vi "Autonomous Independent.vi"() -> ()   [LabVIEW 2013]
doc: "This VI is called when autonomous begins, and will automatically be terminated when autonomous ends. You can carry out timed or sensor driven robot movement independently without needing to return to the caller."
uses:
  <vilib>/Rock Robotics/WPI/Joystick/WPI_JoystickAxis.ctl
  Robot Global Data.vi
  <vilib>/Rock Robotics/WPI/Joystick/WPI_JoystickGetSetRefNum.vi
  <vilib>/Rock Robotics/WPI/RobotDrive/WPI_RobotDriveArcadeDrive_Standard(NoSaturation).vi
panel:
  out "Current Movement, for debugging":T1 {"Y Joystick Value" scale=1.0..-1.0; "X Joystick Value" scale=-1.0..1.0}
  in  "Array of robot movements":T2(array[cluster]) {"Y Joystick Value" scale=1.0..-1.0; "X Joystick Value" scale=-1.0..1.0}
  # "Be sure to right-click and choose Data Operations>>Make Current Value default if you want to save the array values with the VI"
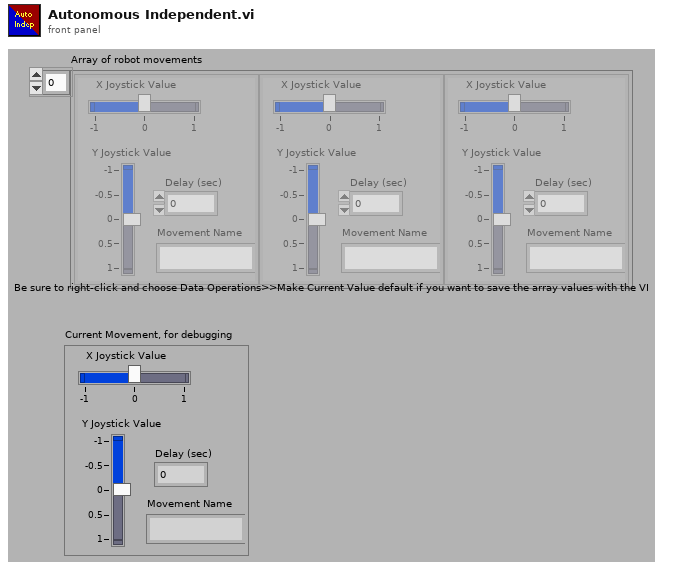
[diagram p1: front panel]
types:
  T1 = cluster{"X Joystick Value":dbl, "Y Joystick Value":dbl, "Delay (sec)":dbl, "Movement Name":string}
  T2 = cluster{"X Joystick Value":dbl, "Y Joystick Value":dbl, "Delay (sec)":dbl, "Movement Name":string}[]
  T3 = typedef "WPI_JoystickAxis.ctl" = enum16{"Axis 1", "Axis 2", "Axis 3", "Axis 4", "Axis 5", "Axis 6"}
  T4 = typedef "WPI_JoystickDevRef.ctl" = cluster{"Device":T5}
  T5 = typedef "WPI_JoystickDeviceEnum.ctl" = enum16{"USB 1", "USB 2", "USB 3", "USB 4", "Kinect 1", "Kinect 2"}
  T6 = typedef "WPI_ServoDeviceRef.ctl" = cluster{"DeviceStatus":errorcluster, "Digital Module":T7, "PWM Channel":T8, "DeadBand":T9}
  T7 = typedef "FPGA_TypedefDigitalModule.ctl" = enum16{"Digital Module 1", "Digital Module 2"}
  T8 = typedef "FPGA_DIOPWMChannel.ctl" = enum8{"PWM 1", "PWM 2", "PWM 3", "PWM 4", "PWM 5", "PWM 6", "PWM 7", "PWM 8", "PWM 9", "PWM 10", "Invalid"}
  T9 = typedef "WPI_PWMDeadband.ctl" = cluster{"Name":string, "maxPositivePwm":i32, "minPositivePwm":i32, "centerPwm":i32, "maxNegativePwm":i32, "minNegativePwm":i32, "angularRange":u16}
  T10 = typedef "WPI_MotorControlDeviceRef.ctl" = cluster{"DeviceStatus":errorcluster, "Type":enum16{"PWM", "CAN"}, "PWM":cluster{"Digital Module":T7, "PWM Channel":T8, "DeadBand":T9}, "CAN":cluster{"Device Number":u8, "Control Mode":T11, "Semaphore":T12, "Max Vout":dbl}, "Invert":bool, "TransformRef":T13, "InvTransformRef":T13}
  T11 = typedef "WPI_CANJaguar_ControlMode.ctl" = enum8{"Percent VBus", "Current", "Speed", "Position", "Voltage"}
  T12 = typedef "Semaphore RefNum" = refnum<k1>
  T13 = typedef "WPI_PWMTransform_ConPane.ctl" = refnum<vi>
  T14 = typedef "WPI_RobotDriveDevRef.ctl" = cluster{"DevStatus":errorcluster, "Motors[]":T10[], "Square Inputs":bool, "Max Output":dbl, "Isochronous":bool}
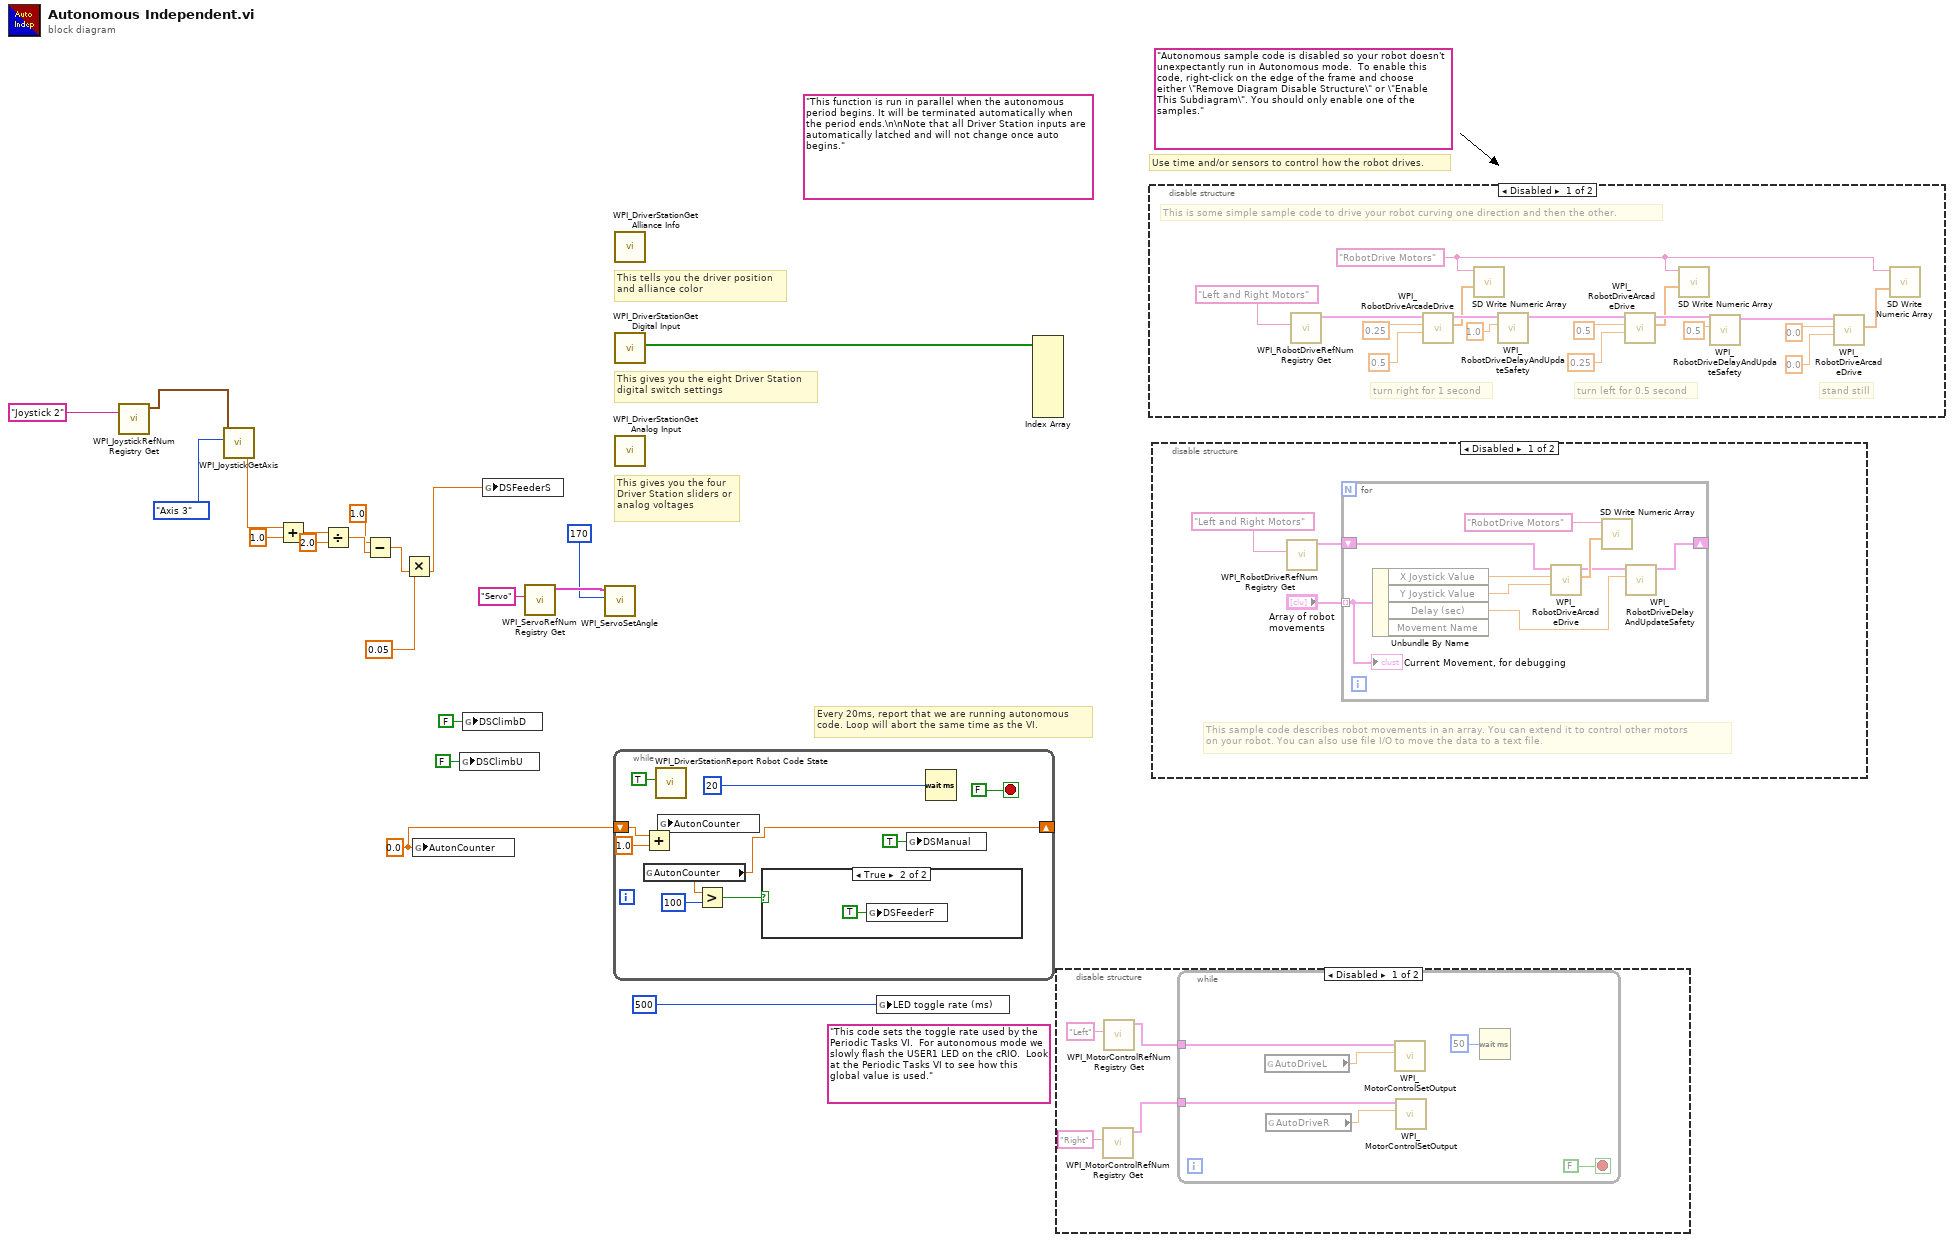
[diagram p0: block diagram]
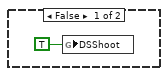
[diagram p5: hidden frame]
diagram:
  w13 = 0.0 ("AutonCounter")
  (unwired) "This code sets the toggle rate used by the Periodic Tasks VI.  For autonomous mode we slowly flash the USER1 LED on the cRIO.  Look at the Periodic Tasks VI to see how this global value is used."
  (unwired) "Autonomous sample code is disabled so your robot doesn't unexpectantly run in Autonomous mode.  To enable this code, right-click on the edge of the frame and choose either \"Remove Diagram Disable Structure\" or \"Enable This Subdiagram\". You should only enable one of the samples."
  (unwired) "This function is run in parallel when the autonomous period begins. It will be terminated automatically when the period ends.\n\nNote that all Driver Station inputs are automatically latched and will not change once auto begins."
  # "Every 20ms, report that we are running autonomous\ncode. Loop will abort the same time as the VI."
  # "Use time and/or sensors to control how the robot drives."
  # "This tells you the driver position\nand alliance color"
  # "This gives you the eight Driver Station\ndigital switch settings"
  # "This gives you the four\nDriver Station sliders or\nanalog voltages"
  n1 = call <vilib>:"WPI_JoystickRefNum Registry Get.vi"("refnum name"="Joystick 2") -> ("JoystickDevRef"=w10:T4)  [unwired: 9 in, 1 out]
  n2 = call <vilib>:"WPI_JoystickGetAxis.vi"("Axis"=WPI_JoystickAxis."Axis 3", "JoystickDevRef"=w10) -> ("Value"=w8:dbl)  [unwired: 8 in, 1 out]
  n3 = Add(x=w8, y=1.0) -> (x+y=w4:dbl)
  n4 = Divide(x=w4, y=2.0) -> (x/y=w2:dbl)
  n5 = Subtract(x=1.0, y=w2) -> (x-y=w12:dbl)
  n6 = Multiply(x=0.05, y=w12) -> (x*y=w7:dbl)
  n7 = global write "Robot Global Data.vi" "AutonCounter"(w13) -> ()
  n8 = global write "Robot Global Data.vi" "DSClimbU"(FALSE ("DSManual")) -> ()
  n9 = global write "Robot Global Data.vi" "DSClimbD"(FALSE ("DSManual")) -> ()
  n10 = global write "Robot Global Data.vi" "DSFeederS"(w7) -> ()
  n11 = call <vilib>:"WPI_ServoRefNum Registry Get.vi"("refnum name"="Servo") -> ("ServoDeviceRef"=w16:T6)  [unwired: 9 in, 1 out]
  n12 = call <vilib>:"WPI_ServoSetAngle.vi"("Angle"=170, "ServoDeviceRef"=w16) -> ()  [unwired: 8 in, 2 out]
  n13 = while {
    shift-right: [w24] -> _
    shift-left: w13 -> [w23]
    stop <- FALSE stop-if-true
    n14 = Add(x=w23, y=1.0) -> (x+y=w21:dbl)
    n15 = global read "Robot Global Data.vi" "AutonCounter"() -> (w24:dbl)
    n16 = call <vilib>:"WPI_DriverStationReport Robot Code State.vi"("Autonomous"=TRUE) -> ()  [unwired: 10 in, 1 out]
    n17 = global write "Robot Global Data.vi" "AutonCounter"(w21) -> ()
    n18 = Greater?(x=w24, y=100) -> (0:w25:bool)
    n19 = case shown="True" w25 {
      frame False {
        n20 = global write "Robot Global Data.vi" "DSShoot"(TRUE ("DSManual")) -> ()
      }
      frame True {
        n21 = global write "Robot Global Data.vi" "DSFeederF"(TRUE ("DSFeederF")) -> ()
      }
    }
    n22 = global write "Robot Global Data.vi" "DSManual"(TRUE ("DSManual")) -> ()
    n23 = Wait (ms)(milliseconds to wait=u32 20) -> ()  [unwired: 1 out]
  }
  n24 = call <vilib>:"WPI_DriverStationGet Alliance Info.vi"() -> ()  [unwired: 12 out]
  n25 = call <vilib>:"WPI_DriverStationGet Digital Input.vi"() -> ("Driver Station Digital Input (1-8)"=w20:bool[])  [unwired: 11 out]
  n26 = call <vilib>:"WPI_DriverStationGet Analog Input.vi"() -> ()  [unwired: 12 out]
  n27 = global write "Robot Global Data.vi" "LED toggle rate (ms)"(u32 500 ("LED ms toggle rate")) -> ()
  n28 = Index Array(array=w20) -> ()  [unwired: 8 in, 8 out]
  n29 = disable-structure shown="Disabled" {
    frame Disabled {
      n30 = call <vilib>:"WPI_MotorControlRefNum Registry Get.vi"("refnum name"="Right") -> ("MotorControlDevRef"=w33:T10)  [unwired: 9 in, 1 out]
      n31 = call <vilib>:"WPI_MotorControlRefNum Registry Get.vi"("refnum name"="Left") -> ("MotorControlDevRef"=w34:T10)  [unwired: 9 in, 1 out]
      n32 = while {
        tunnel: w34 -> [w39]
        tunnel: w33 -> [w38]
        stop <- FALSE stop-if-true
        n33 = global read "Robot Global Data.vi" "AutoDriveL"() -> (w41:dbl)
        n34 = global read "Robot Global Data.vi" "AutoDriveR"() -> (w40:dbl)
        n35 = call <vilib>:"WPI_MotorControlSetOutput.vi"("Output"=w41, "MotorControlDevRef"=w39) -> ()  [unwired: 7 in, 3 out]
        n36 = call <vilib>:"WPI_MotorControlSetOutput.vi"("Output"=w40, "MotorControlDevRef"=w38) -> ()  [unwired: 7 in, 3 out]
        n37 = Wait (ms)(milliseconds to wait=u32 50) -> ()  [unwired: 1 out]
      }
    }
    frame Enabled {
    }
  }
  n38 = disable-structure shown="Disabled" {
    frame Disabled {
      w43 = "RobotDrive Motors" ("Name")
      # "This is some simple sample code to drive your robot curving one direction and then the other."
      # "stand still"
      # "turn left for 0.5 second"
      # "turn right for 1 second"
      n39 = call <vilib>:"WPI_RobotDriveRefNum Registry Get.vi"("refnum name"="Left and Right Motors") -> ("RobotDriveDevRef"=w47:T14)  [unwired: 1 in, 9 out]
      n40 = call-poly <vilib>:"WPI_RobotDriveArcadeDrive.vi"("Y axis value"=0.5 ("X axis value"), "X axis value"=0.25, "RobotDriveDevRef"=w47) -> ("Motor Values"=w46:dbl[], "RobotDriveDevRef"=w54:T14)  [unwired: 1 in, 6 out]
      n41 = call <vilib>:"SD Write Numeric Array.vi"("Numeric Array"=w46, "Name"=w43) -> ()  [unwired: 8 in, 2 out]
      n42 = call <vilib>:"WPI_RobotDriveDelayAndUpdateSafety.vi"("Delay (s)"=1.0, "RobotDriveDevRef"=w54) -> ("RobotDriveDevRef 2"=w53:T14)  [unwired: 8 in, 1 out]
      n43 = call-poly <vilib>:"WPI_RobotDriveArcadeDrive.vi"("Y axis value"=0.25 ("X axis value"), "X axis value"=0.5, "RobotDriveDevRef"=w53) -> ("Motor Values"=w45:dbl[], "RobotDriveDevRef"=w52:T14)  [unwired: 1 in, 6 out]
      n44 = call <vilib>:"SD Write Numeric Array.vi"("Numeric Array"=w45, "Name"=w43) -> ()  [unwired: 8 in, 2 out]
      n45 = call <vilib>:"WPI_RobotDriveDelayAndUpdateSafety.vi"("Delay (s)"=0.5, "RobotDriveDevRef"=w52) -> ("RobotDriveDevRef 2"=w51:T14)  [unwired: 8 in, 1 out]
      n46 = call-poly <vilib>:"WPI_RobotDriveArcadeDrive.vi"("Y axis value"=0.0 ("X axis value"), "X axis value"=0.0, "RobotDriveDevRef"=w51) -> ("Motor Values"=w44:dbl[])  [unwired: 1 in, 7 out]
      n47 = call <vilib>:"SD Write Numeric Array.vi"("Numeric Array"=w44, "Name"=w43) -> ()  [unwired: 8 in, 2 out]
    }
    frame Enabled {
    }
  }
  n48 = disable-structure shown="Disabled" {
    frame Disabled {
      # "This sample code describes robot movements in an array. You can extend it to control other motors\non your robot. You can also use file I/O to move the data to a text file."
      n49 = call <vilib>:"WPI_RobotDriveRefNum Registry Get.vi"("refnum name"="Left and Right Motors") -> ("RobotDriveDevRef"=w62:T14)  [unwired: 1 in, 9 out]
      n50 = for {
        shift-right: [w68] -> _
        shift-left: w62 -> [w69]
        tunnel: "Array of robot movements" -> [w64] mode=indexing
        n51 = Unbundle By Name(w64) -> ("X Joystick Value"=w67:dbl, "Y Joystick Value"=w66:dbl, "Delay (sec)"=w65:dbl)  [unwired: 1 out]
        n52 = call-poly <vilib>:"WPI_RobotDriveArcadeDrive.vi"("Y axis value"=w66, "X axis value"=w67, "RobotDriveDevRef"=w69) -> ("Motor Values"=w71:dbl[], "RobotDriveDevRef"=w70:T14)  [unwired: 1 in, 6 out]
        n53 = call <vilib>:"SD Write Numeric Array.vi"("Numeric Array"=w71, "Name"="RobotDrive Motors") -> ()  [unwired: 8 in, 2 out]
        n54 = call <vilib>:"WPI_RobotDriveDelayAndUpdateSafety.vi"("Delay (s)"=w65, "RobotDriveDevRef"=w70) -> ("RobotDriveDevRef 2"=w68:T14)  [unwired: 8 in, 1 out]
        "Current Movement, for debugging" <- w64
      }
    }
    frame Enabled {
    }
  }
